vi "Tick Count (U64) Global.vi"() -> ()   [LabVIEW 2015]
panel:
  in  "Tick Count Stop":bool
  out "Tick Count (U64)":u64
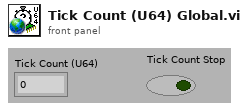
[diagram p1: front panel]
diagram:
